vi "Pane Height.vi"(11 "Panel VI in":refnum<vi>) -> (3 "Panel VI":refnum<vi>, 5 "Height":u32)   [LabVIEW 2020, in "OOPanel.lvlib" / "ArrayManager.lvclass"]
uses:
  ArrayManager.lvclass
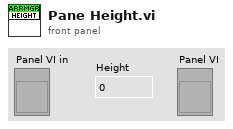
[diagram p1: front panel]
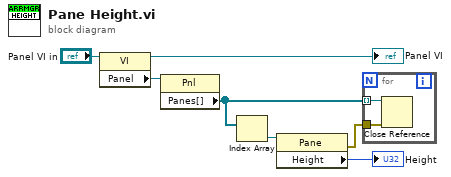
[diagram p0: block diagram]
diagram:
  n1 = property class="VI"(reference="Panel VI in") -> (reference out=→"Panel VI":refnum<vi>, "Panel"=w7:refnum<vi>)  [unwired: 1 in, 1 out]
  n2 = property class="Pnl"(reference=w7) -> ("Panes[]"=w2:refnum<vi>[])  [unwired: 1 in, 2 out]
  n3 = Index Array(array=w2) -> (element=w6:refnum<vi>)  [unwired: 1 in]
  n4 = property class="Pane"(reference=w6) -> (error out=w3:errorcluster, "Height"=→"Height":u32)  [unwired: 1 in, 1 out]
  n5 = for {
    tunnel: w3 -> [w9]
    tunnel: w2 -> [w8] mode=indexing
    n6 = Close Reference(reference=w8, error in (no error)=w9) -> ()  [unwired: 1 out]
  }
